vi "TIO Stream Open.vi"(7 "Port timeout":u32=500, 10 "Default baud":u32=115200, 11 "URL":refnum<visa-resource-name>="tcp://localhost") -> (0 "error out":errorcluster, 1 "Connected":bool=TRUE, 3 "TS Connection":T1={"Type"=enum."TCP", "URL"="serial:///dev/cu.usbserial-00000", "TCP"=refnum, "Timeout"=500, "Route"=""})   [LabVIEW 2017]
uses:
  <vilib>/Instr/_visa.llb/VISA Configure Serial Port (Instr).vi
  <instrlib>/tio-labview/TIO Library/TIO Serial Port Discovery.vi
panel:
  in  "Default Port":i32=7855
  in  "error in (no error)":errorcluster
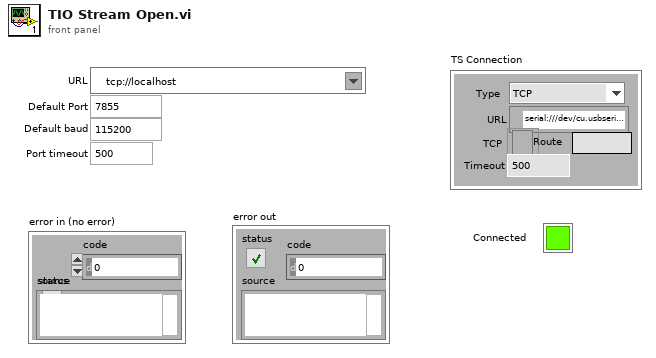
[diagram p1: front panel]
types:
  T1 = cluster{"Type":enum16{"TCP", "Serial"}, "URL":refnum<visa-resource-name>, "TCP":refnum<k5>, "Timeout":u32, "Route":string}
  T2 = cluster{"Type":u16, "VISA resource name out":refnum<visa-resource-name>, "connection ID":refnum<k5>, "Port timeout":u32, "string":string}
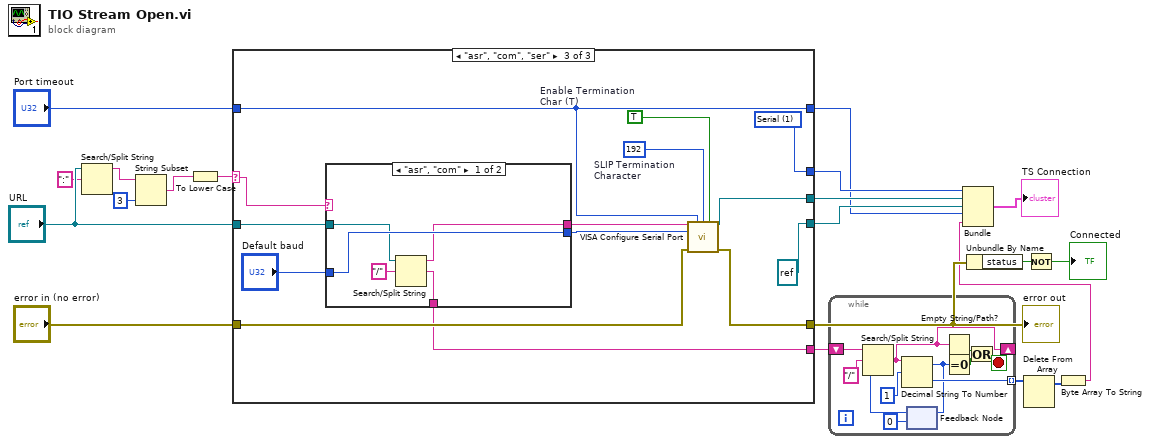
[diagram p0: block diagram]
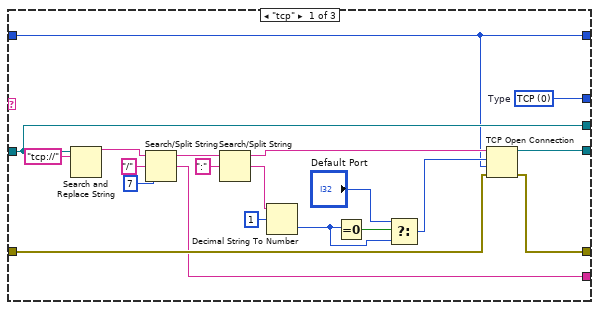
[diagram p2: hidden frame]
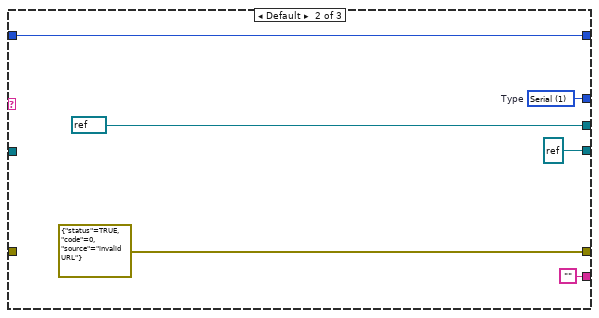
[diagram p3: hidden frame]
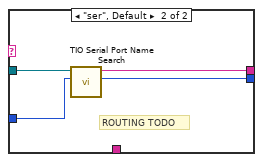
[diagram p4: hidden frame]
diagram:
  n1 = Search/Split String(string="URL", search string/char (-)=":") -> (substring before match=w18:string)  [unwired: 1 in, 2 out]
  n2 = String Subset(string=w18, length (rest)=3 ("length (rest)")) -> (substring=w15:string)  [unwired: 1 in]
  n3 = To Lower Case(string=w15) -> (all lower case string=w16:string)
  n4 = case shown="\"asr\", \"com\", \"ser\"" w16 {
    selector: w16 -> [_ _ w55]
    tunnel: [w31 errorcluster {"status"=TRUE, "code"=0, "source"="invalid URL"} ("error out") w54] -> w14
    tunnel: [w29 refnum<visa-resource-name> refnum ("VISA resource name out") w53] -> w9
    tunnel: "URL" -> [w29 _ w58]
    tunnel: "error in (no error)" -> [w32 _ w52]
    tunnel: [w30 refnum<k5> refnum ("connection ID") refnum<k5> refnum ("connection ID")] -> w8
    tunnel: [w28 w44 w50] -> w11
    tunnel: "Port timeout" -> [w26 w42 w48]
    tunnel: [w26 w42 w48] -> w5
    tunnel: [w21 "" w47] -> w4
    frame "tcp" {
      w28 = u16 0 items=["TCP", "Serial"]  # Type
      n5 = Search and Replace String(input string=w29, search string="tcp://") -> (result string=w23:string)  [unwired: 6 in, 3 out]
      n6 = Search/Split String(string=w23, search string/char (-)="/", offset (0)=7) -> (substring before match=w22:string, match + rest of string=w21:string)  [unwired: 1 out]
      n7 = Search/Split String(string=w22, search string/char (-)=":") -> (substring before match=w33:string, match + rest of string=w38:string)  [unwired: 1 in, 1 out]
      n8 = Decimal String To Number(string=w38, offset=1) -> (number=w36:i32)  [unwired: 1 in, 1 out]
      n9 = Equal To 0?(x=w36) -> (x = 0?=w35:bool)
      n10 = Select(t="Default Port", s=w35, f=w36) -> (s? t:f=w27:i32)
      n11 = TCP Open Connection(address=w33, remote port or service name=w27, timeout ms (60000)=w26, error in (no error)=w32) -> (connection ID=w30:refnum<k5>, error out=w31:errorcluster)  [unwired: 1 in]
    }
    frame Default {
      w44 = u16 1 items=["TCP", "Serial"]  # Type
    }
    frame "asr", "com", "ser" {
      w50 = u16 1 items=["TCP", "Serial"] ("Type")
      w59 = TRUE  # Enable Termination Char (T)
      w60 = u8 192  # SLIP Termination Character
      n12 = case shown="\"asr\", \"com\"" w55 {
        tunnel: w58 -> [w62 w69]
        tunnel: [w61 w68] -> w57
        tunnel: [w65 w67] -> w56
        tunnel: "Default baud" -> [w65 w66]
        tunnel: [w63 _] -> w47
        frame "asr", "com" {
          n13 = Search/Split String(string=w62, search string/char (-)="/") -> (substring before match=w61:string, match + rest of string=w63:string)  [unwired: 1 in, 1 out]
        }
        frame "ser", Default {
          # "ROUTING TODO"
          n14 = call <instrlib>:"TIO Serial Port Name Search.vi"("Default baud"=w66, "String"=w69) -> ("Baud"=w67:i32, "VISA Resource"=w68:string)  [unwired: 7 in, 1 out]
        }
      }
      n15 = call-poly "VISA Configure Serial Port"("VISA resource name"=w57, "timeout (10sec)"=w48, "termination char\n(0xA = '\\n' = LF)"=w60, "Enable Termination\nChar (T)"=w59, "baud rate (9600)"=w56, "error in (no error)"=w52) -> ("VISA resource name out"=w53:refnum<visa-resource-name>, "error out"=w54:errorcluster)  [unwired: 8 in]
    }
  }
  "error out" <- w14
  n16 = while {
    tunnel: [w77] -> w2 mode=indexing
    shift-right: [w73] -> _
    shift-left: w4 -> [w79]
    stop <- w74 stop-if-true
    n17 = feedback #1(0 ("offset past number")) -> (w71:i32)
    n18 = Search/Split String(string=w79, search string/char (-)="/", offset (0)=w71) -> (match + rest of string=w73:string)  [unwired: 2 out]
    n19 = Decimal String To Number(string=w73, offset=1) -> (offset past number=w72:i32, number=w77:i32)  [unwired: 1 in]
    n20 = feedback-in #1(w72) -> ()
    n21 = Empty String/Path?(string/path=w73) -> (empty?=w76:bool)
    n22 = Equal To 0?(x=w72) -> (x = 0?=w75:bool)
    n23 = Or(x=w76, y=w75) -> (x .or. y?=w74:bool)
  }
  n24 = Unbundle By Name(w14) -> ("status"=w13:bool)
  n25 = Delete From Array(array=w2) -> (array with subset deleted=w1:i32[])  [unwired: 2 in, 1 out]
  n26 = Not(x=w13) -> (.not. x?=→"Connected":bool)
  n27 = Byte Array To String(unsigned byte array=w1) -> (string=w3:string)
  n28 = Bundle("Type"=w11, "VISA resource name out"=w9, "connection ID"=w8, "Port timeout"=w5, "string"=w3) -> (→"TS Connection":T2)  [unwired: 1 in]
